vi "Y16byDeviceXML.vi"() -> ()   [LabVIEW 2010]
panel:
  out "error out":errorcluster
  in  "stop":bool
  in  "ICImagingControl":refnum<k7>(container)
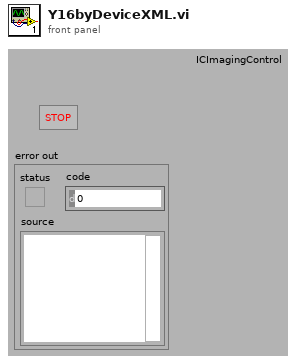
[diagram p1: front panel]
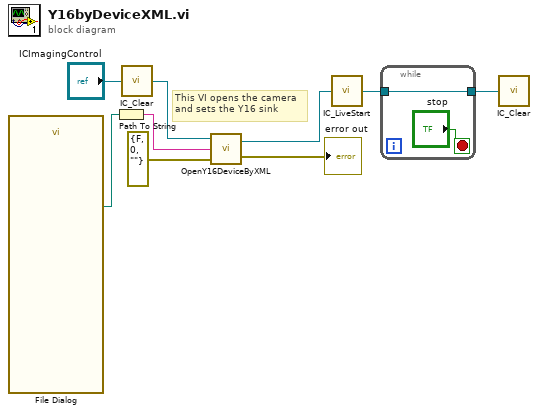
[diagram p0: block diagram]
diagram:
  # "This VI opens the camera\nand sets the Y16 sink"
  n1 = call "File Dialog"() -> ("selected path"=w4:path)  [unwired: 12 in, 3 out]
  n2 = Path To String(path=w4) -> (string=w1:string)
  n3 = call <userlib>:"IC_Clear.vi"("ICImagingControl 2"="ICImagingControl") -> ("ICImagingControl"=w2:refnum<k7>)
  n4 = call <userlib>:"OpenY16DeviceByXML.vi"("error in (no error)"=errorcluster {"status"=FALSE, "code"=0, "source"=""}, "Filename"=w1, "ICImagingControl"=w2) -> ("error out"=→"error out":errorcluster, "ICImagingControl 2"=w9:refnum<k7>)
  n5 = call <userlib>:"IC_LiveStart.vi"("ICImagingControl 3"=w9) -> ("ICImagingControl 2"=w8:refnum<k7>)
  n6 = while {
    tunnel: w8 -> [w10]
    tunnel: [w10] -> w7
    stop <- "stop" stop-if-true
  }
  n7 = call <userlib>:"IC_Clear.vi"("ICImagingControl 2"=w7) -> ()  [unwired: 1 out]
